vi "Retrieve Root Actor.vi"(8 "error in (no error)":errorcluster, 11 "Actor Store in":refnum<class "Actor Store.lvclass">) -> (0 "error out":errorcluster, 1 "valid?":bool, 2 "Root Actor":path, 3 "Actor Store out":refnum<class "Actor Store.lvclass">)   [LabVIEW 2020, in "Add Actor.lvlib" / "Actor Store.lvclass"]
uses:
  Actor Store.lvclass
  Actor Store.lvclass/Actor Store.ctl
  <vilib>/ErrorRing/Error Ring.xnode
  <vilib>/Utility/error.llb/Error Cluster From Error Code.vi
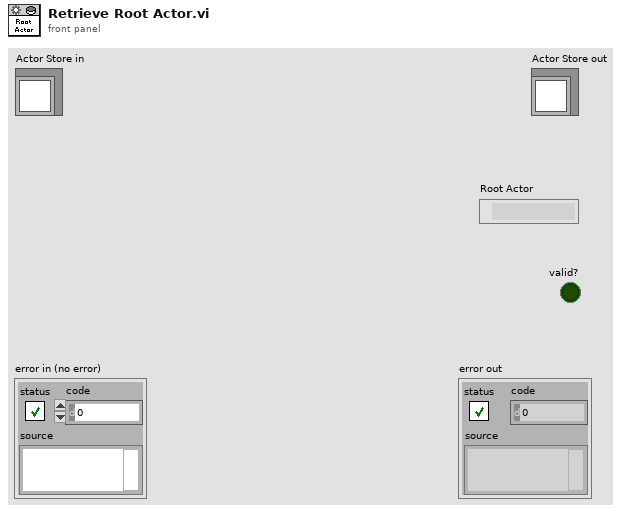
[diagram p1: front panel]
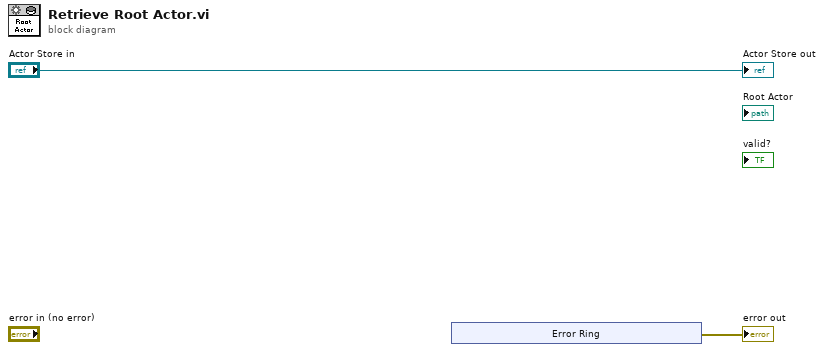
[diagram p0: block diagram]
diagram:
  n1 = xnode "Error Ring"() -> ("error out"=→"error out":errorcluster)
  "Actor Store out" <- "Actor Store in"
